vi "Set.vi"(8 "error in (no error)":errorcluster, 11 "Conrol Value[]":T1[](array[typedef])) -> (0 "error out":errorcluster, 3 "DataObject out":refnum<class "DataObject.lvclass">)   [LabVIEW 2015, in "UndoLibrary.lvlib" / "DataObject.lvclass"]
uses:
  DataObject.lvclass
  Controls/cluster_Control Value.ctl
  DataObject.lvclass/DataObject.ctl
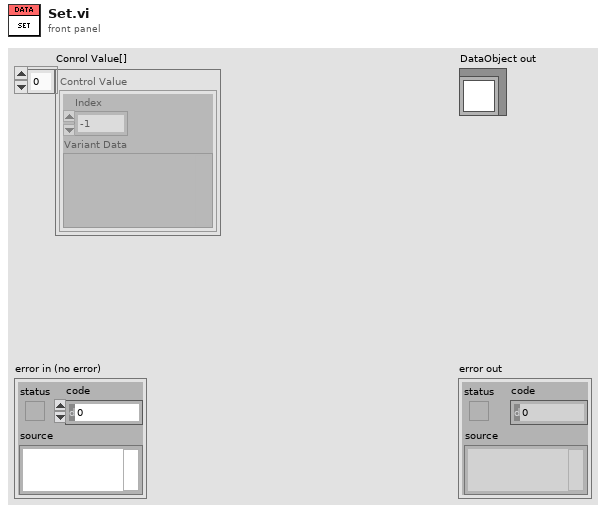
[diagram p1: front panel]
types:
  T1 = typedef "UndoLibrary.lvlib/DataObject.lvclass/cluster_Control Value.ctl" = cluster{"Index":i32, "Variant Data":variant}
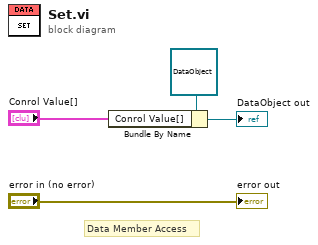
[diagram p0: block diagram]
diagram:
  # "Data Member Access"
  n1 = Bundle By Name(cluster=refnum<class "DataObject.lvclass"> refnum ("UndoLibrary.lvlib:DataObject.lvclass"), "Conrol Value[]"="Conrol Value[]") -> (→"DataObject out":refnum<class "DataObject.lvclass">)
  "error out" <- "error in (no error)"
